vi "sv_Get Actual Max Order.vi"(9 "max order":dbl, 10 "pulse/revolution (1)":i32=1) -> (1 "new pulse/revolution":dbl, 3 "interpolation factor":i32)   [LabVIEW 2017, in "SoundVib_Resampling.lvlib"]
uses:
  <vilib>/addons/Sound and Vibration/Order Analysis/Resample Order Tracking/SoundVib_Resampling.lvlib
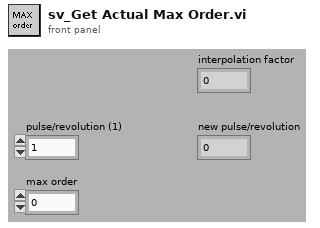
[diagram p1: front panel]
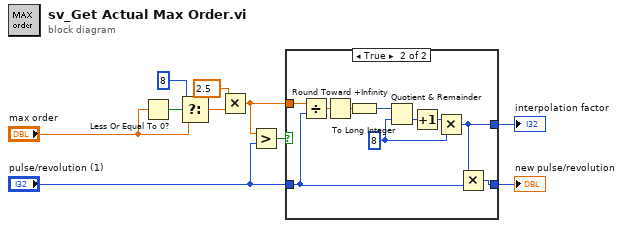
[diagram p0: block diagram]
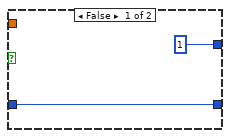
[diagram p2: hidden frame]
diagram:
  n1 = Less Or Equal To 0?(x="max order") -> (x <= 0?=w7:bool)
  n2 = Select(t=8 ("lower limit"), s=w7, f="max order") -> (s? t:f=w9:dbl)
  n3 = Multiply(x=2.5, y=w9) -> (x*y=w5:dbl)
  n4 = Greater?(x=w5, y="pulse/revolution (1)") -> (0:w6:bool)
  n5 = case shown="True" w6 {
    tunnel: w5 -> [_ w22]
    tunnel: "pulse/revolution (1)" -> [w11 w13]
    tunnel: [1 w14] -> w3
    tunnel: [w11 w15] -> w2
    frame False {
    }
    frame True {
      w21 = 8 ("y")
      n6 = Divide(x=w22, y=w13) -> (x/y=w18:dbl)
      n7 = Round Toward +Infinity(x=w18) -> (ceil(x): smallest int >= x=w17:dbl)
      n8 = To Long Integer(number=w17) -> (32bit integer=w16:i32)
      n9 = Quotient & Remainder(x=w16, y=w21) -> (floor(x/y)=w19:i32)  [unwired: 1 out]
      n10 = Increment(x=w19) -> (x+1=w20:i32)
      n11 = Multiply(x=w20, y=w21) -> (x*y=w14:i32)
      n12 = Multiply(x=w14, y=w13) -> (x*y=w15:i32)
    }
  }
  "interpolation factor" <- w3
  "new pulse/revolution" <- w2
